vi "Write Binary File.vi"(8 "error in (no error)":errorcluster, 10 "Data In":dbl[](array[numeric]), 11 "Path":path) -> (0 "error out":errorcluster)   [LabVIEW 2022 SP3]
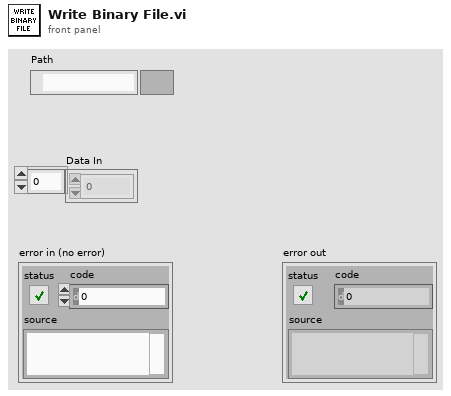
[diagram p1: front panel]
types:
  T1 = enum16{"open", "replace", "create", "open or create", "replace or create", "replace or create with confirmation"}
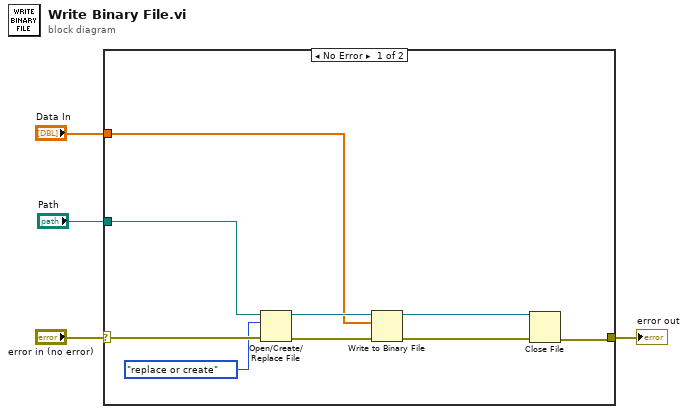
[diagram p0: block diagram]
diagram:
  n1 = case shown="No Error" "error in (no error)" {
    selector: "error in (no error)" -> [w11 w14]
    tunnel: [w12 w14] -> w3
    tunnel: "Path" -> [w13 _]
    tunnel: "Data In" -> [w6 _]
    frame No Error {
      n2 = Open/Create/Replace File(file path (use dialog)=w13, error in=w11, operation (0:open)=T1."replace or create") -> (refnum out=w8:refnum<file>, error out=w10:errorcluster)  [unwired: 3 in, 1 out]
      n3 = Write to Binary File(file (use dialog)=w8, data=w6, error in=w10) -> (refnum out=w7:refnum<file>, error out=w9:errorcluster)  [unwired: 3 in, 1 out]
      n4 = Close File(refnum=w7, error in=w9) -> (error out=w12:errorcluster)  [unwired: 1 out]
    }
    frame Error {
    }
  }
  "error out" <- w3
